vi "_Start Monitor VI.vi"(8 "error in (no error)":errorcluster) -> (0 "error out":errorcluster)   [LabVIEW 2014, in "TagDB(dev).lvlib"]
uses:
  TagDB(dev).lvlib
  _Monitor.vi
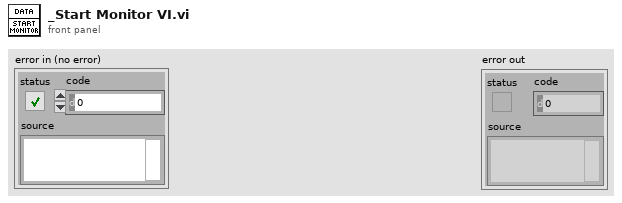
[diagram p1: front panel]
types:
  T1 = enum32{"Bad", "Idle", "Run top level", "Running"}
  T2 = enum32{"Invalid", "Standard", "Closed", "Hidden", "Minimized", "Maximized"}
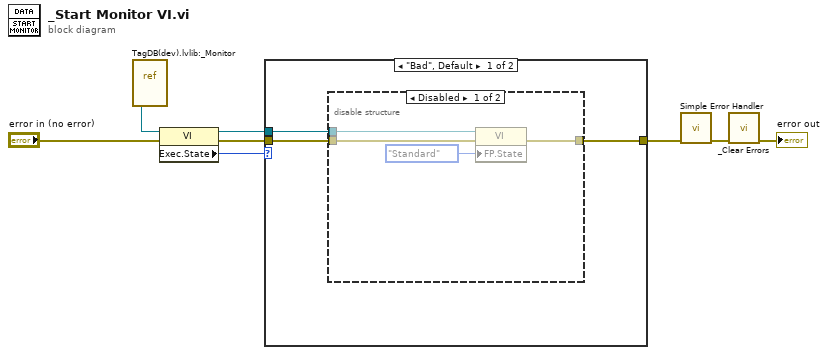
[diagram p0: block diagram]
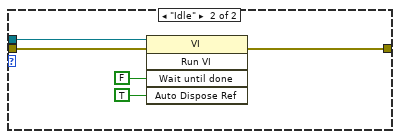
[diagram p3: hidden frame]
diagram:
  n1 = vi-ref "TagDB(dev).lvlib:_Monitor.vi"() -> (w8:refnum<vi>)
  n2 = property class="VI"(reference=w8, error in="error in (no error)") -> (reference out=w5:refnum<vi>, error out=w7:errorcluster, "Exec.State"=w6:T1)
  n3 = case shown="\"Bad\", Default" w6 {
    tunnel: w7 -> [w11 w20]
    tunnel: w5 -> [w9 w21]
    tunnel: [w10 w17] -> w4
    frame "Bad", Default {
      n4 = disable-structure shown="Disabled" {
        disable-tunnel: w11 -> [w15 w16]
        disable-tunnel: [w14 w16] -> w10
        disable-tunnel: w9 -> [w13 _]
        frame Disabled {
          n5 = property class="VI"(reference=w13, error in=w15, "FP.State"=T2."Standard" ("Front Panel Window:State")) -> (error out=w14:errorcluster)  [unwired: 1 out]
        }
        frame Enabled {
        }
      }
    }
    frame "Idle" {
      n6 = invoke class="VI" method="Run VI"(reference=w21, error in=w20, "Wait until done"=FALSE ("Wait Until Done"), "Auto Dispose Ref"=TRUE ("Auto Dispose Reference")) -> (error out=w17:errorcluster)  [unwired: 1 in, 4 out]
    }
  }
  n7 = call <vilib>:"Simple Error Handler.vi"("error in (no error)"=w4) -> ("error out"=w3:errorcluster)  [unwired: 4 in, 4 out]
  n8 = call "_Clear Errors.vi"("error in (no error)"=w3) -> ("error out"=→"error out":errorcluster)  [unwired: 5 in, 1 out]
